vi "remote.Initialize (Remote No Resource).vi"(1 "Hostname/IP":string, 2 "Port":u16, 3 "https?":bool, 11 "error in (no error)":errorcluster, 13 "username":string="admin", 14 "password":string) -> (4 "SLSC Remote out":refnum<class "SLSC Interface.lvclass">, 15 "error out":errorcluster)   [LabVIEW 2016, in "SLSC Interfaces.lvlib" / "SLSC Interface.lvclass"]
uses:
  SLSC Interface Class/SLSC Interface.lvclass
  SLSC Interface Class/slsc type.ctl
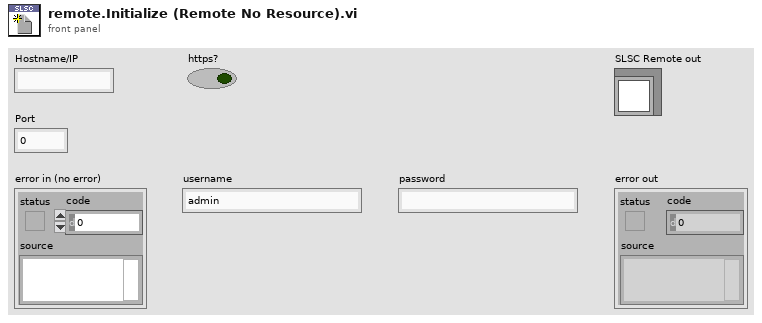
[diagram p1: front panel]
types:
  T1 = typedef "SLSC Interfaces.lvlib/SLSC Interface.lvclass/slsc type.ctl" = enum16{"device", "nvmem", "channel", "none"}
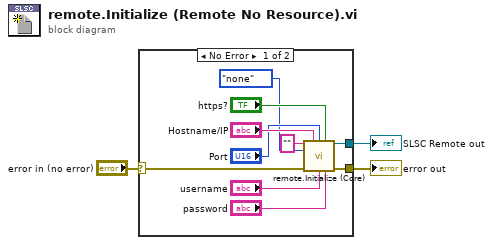
[diagram p0: block diagram]
diagram:
  n1 = case shown="No Error" "error in (no error)" {
    selector: "error in (no error)" -> [w13 w14]
    tunnel: [w11 w14] -> w2
    tunnel: [w12 _] -> w1
    frame No Error {
      n2 = call "remote.Initialize (Core).vi"("resources"="", "Hostname/IP"="Hostname/IP", "Port"="Port", "https?"="https?", "slsc type"=slsc_type."none", "error in (no error)"=w13, "username"="username", "password"="password") -> ("SLSC Remote out"=w12:refnum<class "SLSC Interface.lvclass">, "error out"=w11:errorcluster)  [unwired: 6 in]
    }
    frame Error {
    }
  }
  "error out" <- w2
  "SLSC Remote out" <- w1
